vi "CRC-8.vi"(6 "Reflected":bool, 8 "FinalXorValue":u8 format="%02x", 9 "InitialCRC":u8 format="%02x", 10 "Polynomial":u8 format="%02x", 11 "DATA":u8[](array[numeric]) format="%02x") -> (3 "CRC":u8 format="%02x")   [LabVIEW 2021, in "LIN Frame Protection Addon Engine.lvlib"]
uses:
  LIN Frame Protection Addon Engine.lvlib
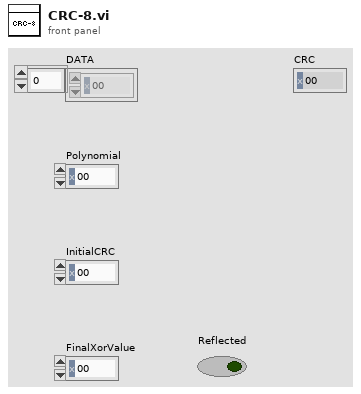
[diagram p1: front panel]
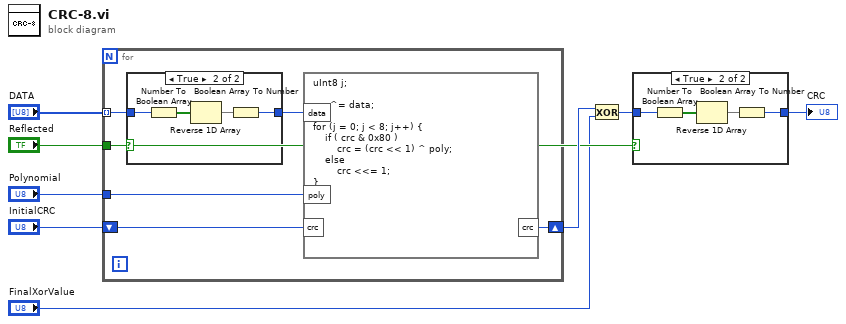
[diagram p0: block diagram]
diagram:
  n1 = for {
    tunnel: "Polynomial" -> [w14]
    tunnel: "DATA" -> [w10] mode=indexing
    tunnel: "Reflected" -> [w12]
    shift-right: [w9] -> w5
    shift-left: "InitialCRC" -> [w13]
    n2 = case shown="True" w12 {
      tunnel: [w15 w18] -> w11
      tunnel: w10 -> [w15 w19]
      frame False {
      }
      frame True {
        n3 = Number To Boolean Array(number=w19) -> (Boolean array=w17:bool[])
        n4 = Reverse 1D Array(array=w17) -> (reversed array=w16:bool[])
        n5 = Boolean Array To Number(Boolean array=w16) -> (number=w18:u8)
      }
    }
    n6 = formula code="uInt8 j;\n\ncrc ^= data;\n\nfor (j = 0; j < 8; j++) {\n    if ( crc & 0x80 )\n        crc = (crc << 1) ^ poly;\n    else\n        crc <<= 1;\n}"("poly"=w14, "data"=w11, "crc"=w13) -> ("crc"=w9:u8)
  }
  n7 = Exclusive Or(1:"FinalXorValue", 2:w5) -> (0:w2:u8)
  n8 = case shown="True" "Reflected" {
    tunnel: [w20 w23] -> w3
    tunnel: w2 -> [w20 w24]
    frame False {
    }
    frame True {
      n9 = Number To Boolean Array(number=w24) -> (Boolean array=w22:bool[])
      n10 = Reverse 1D Array(array=w22) -> (reversed array=w21:bool[])
      n11 = Boolean Array To Number(Boolean array=w21) -> (number=w23:u8)
    }
  }
  "CRC" <- w3
